vi "Serving Coffee.vi"() -> ()   [LabVIEW 2021]
uses:
  Espresso/Espresso.lvclass
  C:/Users/nina/Documents/Head First Design Patterns/HeadFirstDesignPatternsLabVIEWandPython/03 Decorator/LabVIEW/Beverage/Beverage.lvclass
  Mocha/Mocha.lvclass
  Beverage/Beverage.lvclass
panel:
  out "error out":errorcluster
  out "Description":string
  # "Locals"
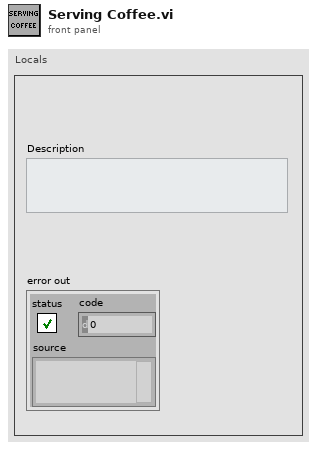
[diagram p1: front panel]
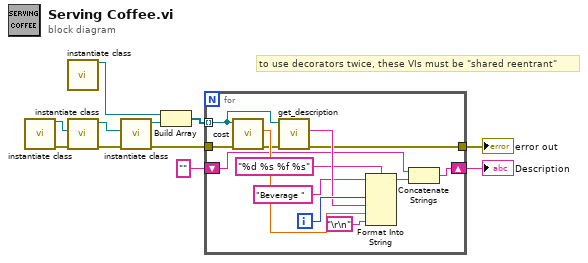
[diagram p0: block diagram]
diagram:
  # "to use decorators twice, these VIs must be \"shared reentrant\""
  n1 = call "instantiate class.vi"() -> ("Espresso"=w9:refnum<class "Espresso.lvclass">, "error out"=w10:errorcluster)  [unwired: 14 in]
  n2 = call "instantiate class.vi"() -> ("Espresso"=w11:refnum<class "Espresso.lvclass">)  [unwired: 14 in, 1 out]
  n3 = call "instantiate class.vi"("error in (no error)"=w10, "Beverage to be wrapped.lvclass"=w9) -> ("error out"=w2:errorcluster, "Mocha out"=w4:refnum<class "Mocha.lvclass">)  [unwired: 8 in]
  n4 = call "instantiate class.vi"("error in (no error)"=w2, "Beverage to be wrapped.lvclass"=w4) -> ("error out"=w1:errorcluster, "Mocha out"=w3:refnum<class "Mocha.lvclass">)  [unwired: 8 in]
  n5 = Build Array(w11, w3) -> (w8:refnum<class "Beverage.lvclass">[])
  n6 = for {
    tunnel: w8 -> [w24] mode=indexing
    shift-right: [w15] -> w6
    shift-left: "" -> [w17]
    tunnel: w1 -> [w14]
    tunnel: [w12] -> w5
    i -> [w23]
    n7 = call-dynamic "cost.vi"("error in (no error)"=w14, "Beverage in"=w24) -> ("error out"=w13:errorcluster, "Cost"=w19:dbl)  [unwired: 7 in, 1 out]
    n8 = call-dynamic "get_description.vi"("error in (no error)"=w13, "Beverage in"=w24) -> ("error out"=w12:errorcluster, "Description"=w22:string)  [unwired: 7 in, 1 out]
    n9 = Format Into String(format string="%d %s %f %s", initial string="Beverage ", w23, w22, w19, "\r\n") -> (resulting string=w16:string)  [unwired: 1 in, 1 out]
    n10 = Concatenate Strings(w17, w16) -> (w15:string)
  }
  "Description" <- w6
  "error out" <- w5
